vi "Configure Math.vi"(7 "Enable Math Function (T:Enable)":bool=TRUE, 8 "error in (no error)":errorcluster, 9 "Custom Math Operation Name (\"Custom\")":string="Custom", 10 "Math Operation (0: Power)":u16(ring) items=["Power", "Offset Compensated Ohms", "Resistor Voltage Coefficient", "Varistor Alpha", "Custom Math Operation"], 11 "VISA resource name":refnum<visa-resource-name>) -> (0 "error out":errorcluster, 3 "VISA resource name out":refnum<visa-resource-name>)   [LabVIEW 2022 SP3, in "Keithley 24XX.lvlib"]
doc: "Configure the math operation performed by the instrument on collected data."
uses:
  <instrlib>/Keithley 24XX/Keithley 24XX.lvlib
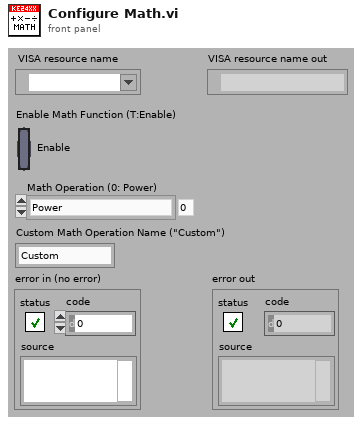
[diagram p1: front panel]
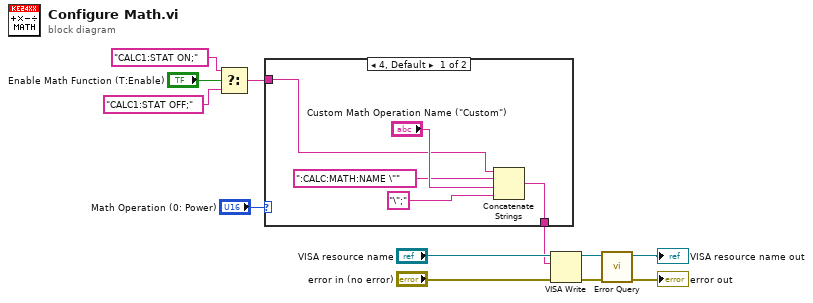
[diagram p0: block diagram]
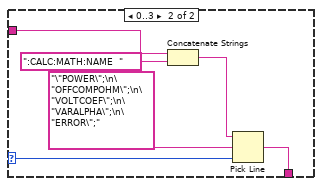
[diagram p2: hidden frame]
diagram:
  n1 = Select(t="CALC1:STAT ON;", s="Enable Math Function (T:Enable)", f="CALC1:STAT OFF;") -> (s? t:f=w1:string)
  n2 = case shown="4, Default" "Math Operation (0: Power)" {
    selector: "Math Operation (0: Power)" -> [_ w21]
    tunnel: [w16 w22] -> w10
    tunnel: w1 -> [w13 w19]
    frame 4, Default {
      n3 = Concatenate Strings(w13, ":CALC:MATH:NAME \"", "Custom Math Operation Name (\"Custom\")", "\";" ("string")) -> (w16:string)
    }
    frame 0..3 {
      n4 = Concatenate Strings(w19, ":CALC:MATH:NAME  " ("string (\"\")")) -> (w18:string)
      n5 = Pick Line(string ("")=w18, multi-line string="\"POWER\";\n\"OFFCOMPOHM\";\n\"VOLTCOEF\";\n\"VARALPHA\";\n\"ERROR\";", line index=w21) -> (output string=w22:string)
    }
  }
  n6 = VISA Write(VISA resource name="VISA resource name", write buffer=w10, error in (no error)="error in (no error)") -> (VISA resource name out=w9:refnum<visa-resource-name>, error out=w6:errorcluster)  [unwired: 1 out]
  n7 = call <instrlib>:"Error Query.vi"("error in (no error)"=w6, "VISA resource name"=w9) -> ("error out"=→"error out":errorcluster, "VISA resource name out"=→"VISA resource name out":refnum<visa-resource-name>)  [unwired: 6 in, 2 out]
